vi "Subpanel UI.vi"(8 "error in (no error)":errorcluster, 10 "Message Queue":refnum<queue>, 11 "Controller in":refnum<class "LC Parser.lvclass">) -> (0 "error out":errorcluster, 3 "Controller out":refnum<class "LC Parser.lvclass">)   [LabVIEW 2020, in "LC Parser.lvclass"]
doc: "Dynamic dispatch VI that must be overridden by all inheriting classes. It is the UI that will be inserted into subpanels so data can be displayed to the user. The class will use an internally managed message queue to communicate to it. The user should only communicate to this UI through class methods."
uses:
  LC Parser.lvclass
  LC Parser.lvclass/LC Parser.ctl
  Controller/Generic Plugin.lvclass
  Sub VIs/Message Queue/Message Cluster.ctl
  Sub VIs/Message Queue/test Message Queue.lvlib
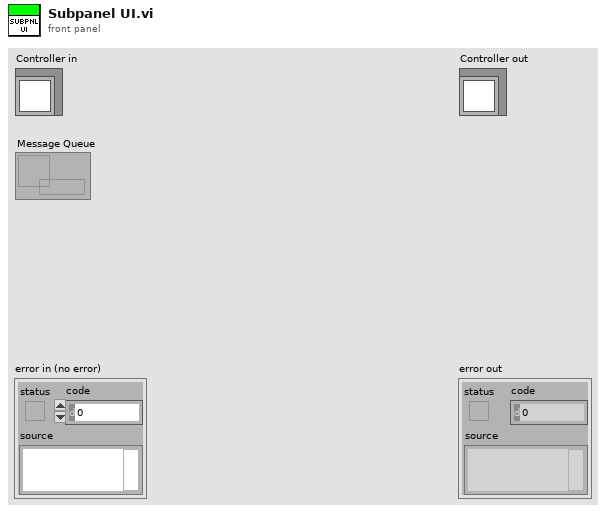
[diagram p1: front panel]
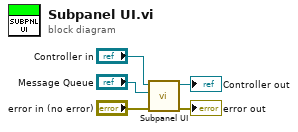
[diagram p0: block diagram]
diagram:
  n1 = call-parent "Subpanel UI.vi"("error in (no error)"="error in (no error)", "Message Queue"="Message Queue", "Controller in"="Controller in") -> ("error out"=→"error out":errorcluster, "Controller out"=→"Controller out":refnum<class "LC Parser.lvclass">)  [unwired: 7 in]
